vi "WarnCheck_Move2Pos_present.vi"(8 "Error In":errorcluster, 11 "Macro Command String IN":string="LOOP.Start\t(loop.iterations,3.000);") -> (0 "Error Out":errorcluster, 3 "Invalid params type?":bool)   [LabVIEW 2012]
doc: "SciScan 1.2 160622"
uses:
  MacroRules_FGV_Commands.ctl
  <vilib>/Utility/error.llb/whitespace.ctl
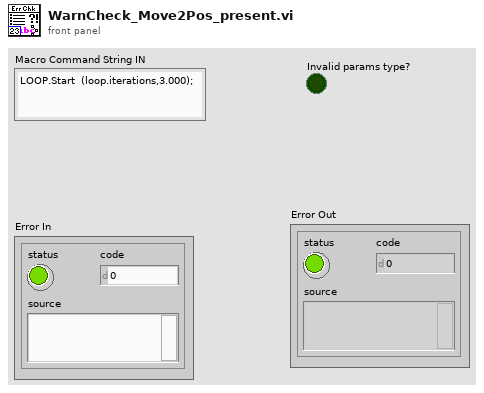
[diagram p1: front panel]
types:
  T1 = typedef "whitespace.ctl" = u16
  T2 = typedef "MacroRules_FGV_Commands.ctl" = enum16{"Read File", "Get All", "Get Param and Flags"}
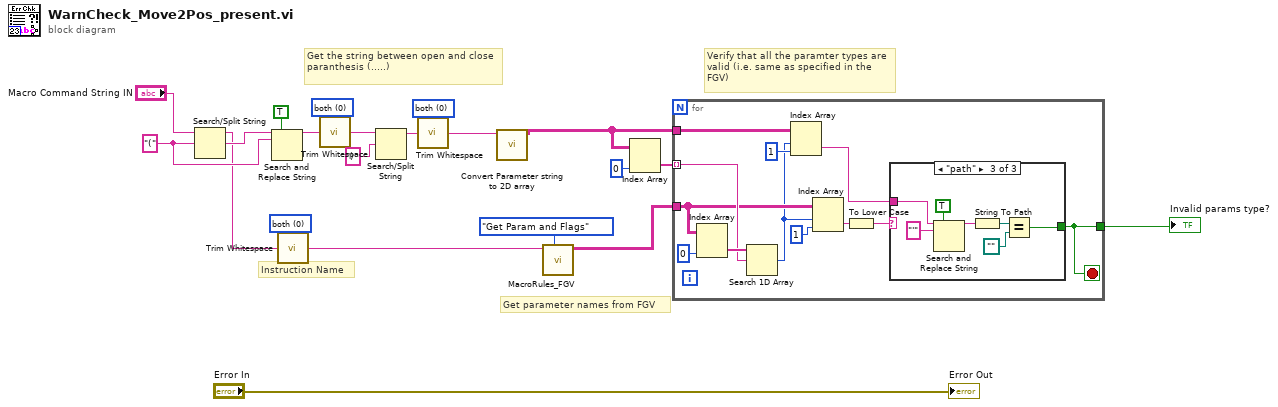
[diagram p0: block diagram]
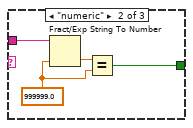
[diagram p3: hidden frame]
diagram:
  w8 = T1 0 items=["both", "start of string", "end of string"] ("location (both)")
  w18 = T1 0 items=["both", "start of string", "end of string"] ("location (both)")
  w21 = T1 0 items=["both", "start of string", "end of string"] ("location (both)")
  w12 = "(" ("search string/char (-)")
  # "Get parameter names from FGV"
  # "Instruction Name"
  # "Verify that all the paramter types are valid (i.e. same as specified in the FGV)"
  # "Get the string between open and close paranthesis (.....)"
  n1 = Search/Split String(string="Macro Command String IN", search string/char (-)=w12) -> (substring before match=w7:string, match + rest of string=w11:string)  [unwired: 1 in, 1 out]
  n2 = Search and Replace String(replace all?=TRUE ("replace all? (F)"), input string=w11, search string=w12) -> (result string=w13:string)  [unwired: 5 in, 3 out]
  n3 = call <vilib>:"Trim Whitespace.vi"("string"=w7, "location (both)"=w8) -> ("trimmed string"=w6:string)
  n4 = call <vilib>:"Trim Whitespace.vi"("string"=w13, "location (both)"=w21) -> ("trimmed string"=w10:string)
  n5 = Search/Split String(string=w10, search string/char (-)=")") -> (substring before match=w19:string)  [unwired: 1 in, 2 out]
  n6 = call <vilib>:"Trim Whitespace.vi"("string"=w19, "location (both)"=w18) -> ("trimmed string"=w9:string)
  n7 = call "Convert Parameter string to 2D array.vi"("Parameter string IN (without paranthesis)"=w9) -> ("Params table OUT"=w3:string[][])  [unwired: 7 in, 3 out]
  n8 = call "MacroRules_FGV.vi"("MacroRules_FGV_Commands"=MacroRules_FGV_Commands."Get Param and Flags", "Command Name IN"=w6) -> ("Parameters"=w2:string[][])  [unwired: 5 in, 4 out]
  n9 = Index Array(array=w3, index (col)=0 ("disabled index (col)")) -> (element=w4:string[])  [unwired: 1 in]
  n10 = for {
    tunnel: w2 -> [w27]
    tunnel: w4 -> [w31] mode=indexing
    tunnel: w3 -> [w30]
    tunnel: [w22] -> w1
    stop <- w22 stop-if-true
    n11 = Index Array(array=w27, index (col)=0 ("disabled index (col)")) -> (element=w32:string[])  [unwired: 1 in]
    n12 = Search 1D Array(1D array=w32, element=w31) -> (index of element=w26:i32)  [unwired: 1 in]
    n13 = Index Array(array=w30, index (row)=w26, index (col)=1 ("disabled index (col)")) -> (element=w23:string)
    n14 = Index Array(array=w27, index (row)=w26, index (col)=1 ("disabled index (col)")) -> (element=w25:string)
    n15 = To Lower Case(string=w25) -> (all lower case string=w24:string)
    n16 = case shown="\"path\"" w24 {
      tunnel: w23 -> [_ w37 w44]
      tunnel: [_ w34 w40] -> w22
      frame Default {
      }
      frame "numeric" {
        w35 = 999999.0 ("default (0 DBL)")
        n17 = Fract/Exp String To Number(string=w37, default (0 dbl)=w35) -> (number=w36:dbl)  [unwired: 2 in, 1 out]
        n18 = Equal?(x=w36, y=w35) -> (x = y?=w34:bool)
      }
      frame "path" {
        n19 = Search and Replace String(replace all?=TRUE ("replace all? (F)"), input string=w44, search string="'") -> (result string=w41:string)  [unwired: 5 in, 3 out]
        n20 = String To Path(string=w41) -> (path=w39:path)
        n21 = Equal?(x=w39, y=path "") -> (x = y?=w40:bool)
      }
    }
  }
  "Invalid params type?" <- w1
  "Error Out" <- "Error In"
